vi "Create RxTx.vi"(8 "error in (no error)":errorcluster, 9 "Python path":string="200.131.64.49", 10 "Remote IP:":string="200.131.64.49", 11 "Channel in":refnum<class "Channel.lvclass">) -> (0 "error out":errorcluster, 3 "Channel out":refnum<class "Channel.lvclass">)   [LabVIEW 2018, in "Channel.lvclass"]
doc: "Create the queres responsible for communication"
uses:
  Channel.lvclass
  Channel.lvclass/Channel.ctl
  RxTx/RxTx.lvclass
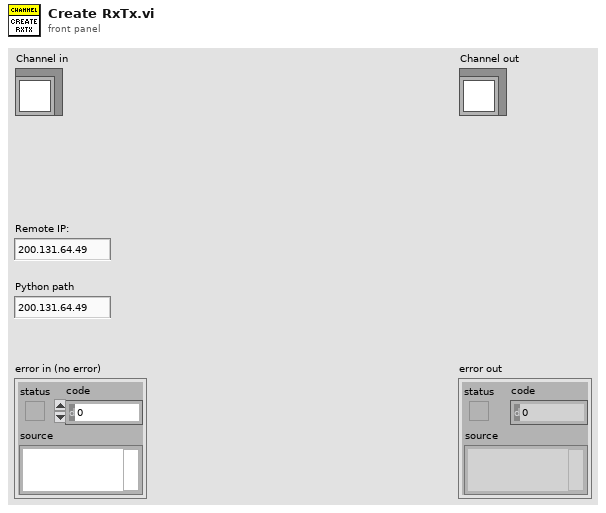
[diagram p1: front panel]
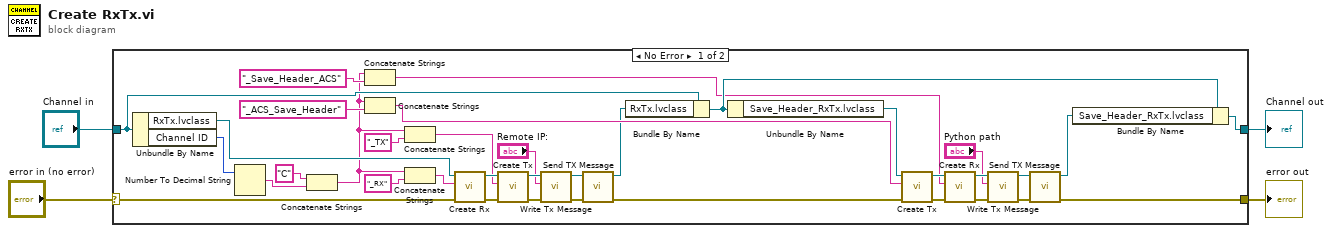
[diagram p0: block diagram]
diagram:
  n1 = case shown="No Error" "error in (no error)" {
    selector: "error in (no error)" -> [w26 w42]
    tunnel: [w24 w42] -> w3
    tunnel: [w27 w41] -> w1
    tunnel: "Channel in" -> [w37 w41]
    frame No Error {
      n2 = Unbundle By Name(w37) -> ("RxTx.lvclass"=w39:refnum<class "RxTx.lvclass">, "Channel ID"=w15:u8)
      n3 = Number To Decimal String(number=w15) -> (decimal integer string=w34:string)  [unwired: 1 in]
      n4 = Concatenate Strings("C", w34) -> (w19:string)
      n5 = Concatenate Strings(w19, "_Save_Header_ACS") -> (w21:string)
      n6 = Concatenate Strings(w19, "_ACS_Save_Header") -> (w18:string)
      n7 = Concatenate Strings(w19, "_TX") -> (w32:string)
      n8 = Concatenate Strings(w19, "_RX") -> (w30:string)
      n9 = call "Create Rx.vi"("error in (no error)"=w26, "Reader Name"=w30, "RxTx in"=w39) -> ("error out"=w40:errorcluster, "RxTx out"=w38:refnum<class "RxTx.lvclass">)  [unwired: 7 in]
      n10 = call "Create Tx.vi"("error in (no error)"=w40, "Writer Name"=w32, "RxTx in"=w38) -> ("error out"=w11:errorcluster, "RxTx out"=w14:refnum<class "RxTx.lvclass">)  [unwired: 7 in]
      n11 = call "Write Tx Message.vi"("error in (no error)"=w11, "Tx Message"="Remote IP:", "RxTx in"=w14) -> ("error out"=w12:errorcluster, "RxTx out"=w13:refnum<class "RxTx.lvclass">)  [unwired: 7 in]
      n12 = call "Send TX Message.vi"("error in (no error)"=w12, "RxTx in"=w13) -> ("error out"=w16:errorcluster, "RxTx out"=w17:refnum<class "RxTx.lvclass">)  [unwired: 8 in]
      n13 = Bundle By Name(cluster=w37, "RxTx.lvclass"=w17) -> (w28:refnum<class "Channel.lvclass">)
      n14 = Unbundle By Name(w28) -> ("Save_Header_RxTx.lvclass"=w36:refnum<class "RxTx.lvclass">)
      n15 = call "Create Tx.vi"("error in (no error)"=w16, "Writer Name"=w18, "RxTx in"=w36) -> ("error out"=w23:errorcluster, "RxTx out"=w22:refnum<class "RxTx.lvclass">)  [unwired: 7 in]
      n16 = call "Create Rx.vi"("error in (no error)"=w23, "Reader Name"=w21, "RxTx in"=w22) -> ("error out"=w6:errorcluster, "RxTx out"=w7:refnum<class "RxTx.lvclass">)  [unwired: 7 in]
      n17 = call "Write Tx Message.vi"("error in (no error)"=w6, "Tx Message"="Python path", "RxTx in"=w7) -> ("error out"=w9:errorcluster, "RxTx out"=w8:refnum<class "RxTx.lvclass">)  [unwired: 7 in]
      n18 = call "Send TX Message.vi"("error in (no error)"=w9, "RxTx in"=w8) -> ("error out"=w24:errorcluster, "RxTx out"=w25:refnum<class "RxTx.lvclass">)  [unwired: 8 in]
      n19 = Bundle By Name(cluster=w28, "Save_Header_RxTx.lvclass"=w25) -> (w27:refnum<class "Channel.lvclass">)
    }
    frame Error {
    }
  }
  "error out" <- w3
  "Channel out" <- w1
